vi "AI_StreamingBufferedRead.vi"(8 "error in (no error)":errorcluster, 10 "stop?":bool, 11 "Task ID":u32) -> (0 "error out":errorcluster, 1 "stopped":bool, 2 "data out":dynamicdata(graph), 3 "Task out ID":u32)   [LabVIEW 2015]
panel:
  out "status":bool
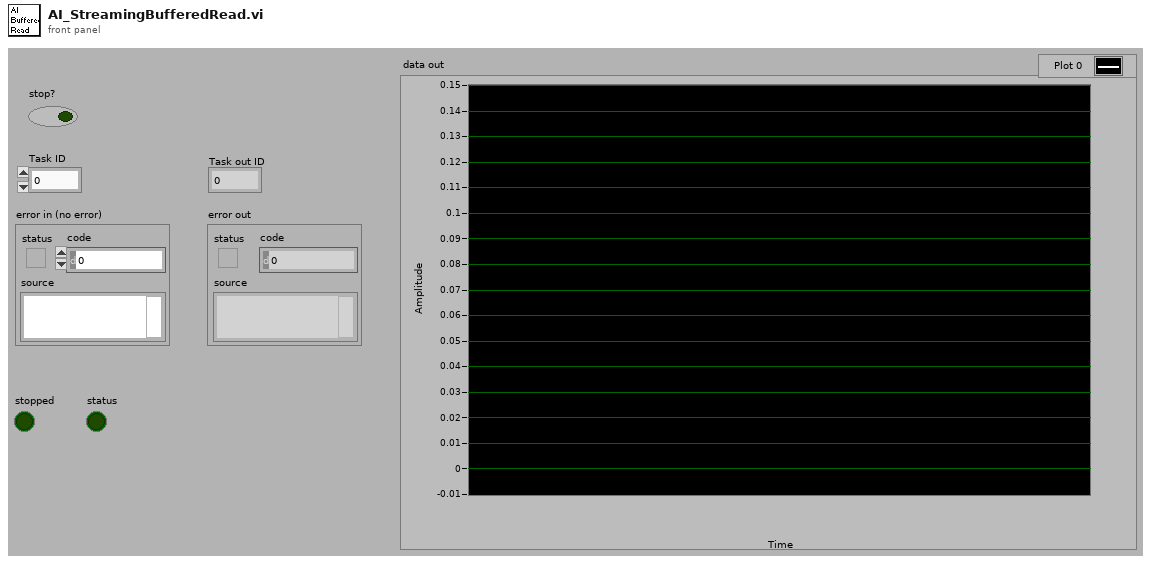
[diagram p1: front panel]
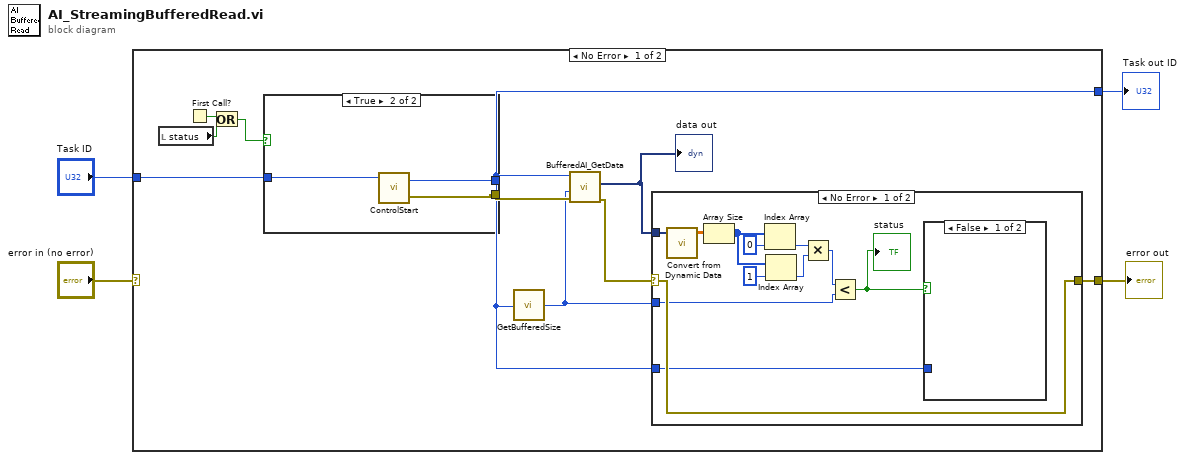
[diagram p0: block diagram]
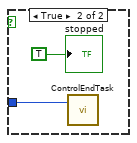
[diagram p2: hidden frame]
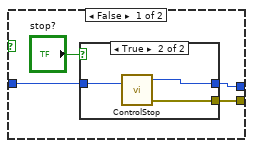
[diagram p4: hidden frame]
diagram:
  n1 = case shown="No Error" "error in (no error)" {
    selector: "error in (no error)" -> [_ w41]
    tunnel: "Task ID" -> [w14 w42]
    tunnel: [w9 w42] -> w2
    tunnel: [w12 w41] -> w1
    frame No Error {
      n2 = local read "status"() -> (w5:bool)
      n3 = First Call?() -> (First Call?: T/F=w7:bool)
      n4 = Or(x=w7, y=w5) -> (x .or. y?=w6:bool)
      n5 = case shown="True" w6 {
        tunnel: w14 -> [w33 w40]
        tunnel: [w31 w39] -> w9
        tunnel: [w30 w38] -> w10
        frame False {
          n6 = case shown="True" "stop?" {
            tunnel: w33 -> [w34 w37]
            tunnel: [w34 w36] -> w31
            tunnel: [_ w35] -> w30
            frame False {
            }
            frame True {
              n7 = call "ControlStop.vi"("Task ID"=w37) -> ("error out"=w35:errorcluster, "Task ID"=w36:u32)  [unwired: 1 in, 2 out]
            }
          }
        }
        frame True {
          n8 = call "ControlStart.vi"("Task ID"=w40) -> ("error out"=w38:errorcluster, "Task ID"=w39:u32)  [unwired: 1 in, 1 out]
        }
      }
      n9 = call "GetBufferedSize.vi"("Task ID"=w9) -> ("return type"=w8:i32)
      n10 = call "BufferedAI_GetData.vi"("error in (no error)"=w10, "count"=w8, "Task ID"=w9) -> ("error out"=w13:errorcluster, "data out"=w11:dynamicdata)  [unwired: 1 in, 6 out]
      "data out" <- w11
      n11 = case shown="No Error" w13 {
        selector: w13 -> [w25 w29]
        tunnel: [w25 w29] -> w12
        tunnel: w11 -> [w26 _]
        tunnel: w9 -> [w24 _]
        tunnel: w8 -> [w16 _]
        frame No Error {
          n12 = call "Convert from Dynamic Data"("Dynamic Data Type"=w26) -> ("Array"=w23:dbl[][])  [unwired: 3 out]
          n13 = Array Size(array=w23) -> (size(s)=w21:i32[])
          n14 = Index Array(array=w21, index=0) -> (element=w18:i32)
          n15 = Index Array(array=w21, index=1) -> (element=w19:i32)
          n16 = Multiply(x=w18, y=w19) -> (x*y=w17:i32)
          n17 = Less?(x=w17, y=w16) -> (x < y?=w15:bool)
          "status" <- w15
          n18 = case shown="False" w15 {
            tunnel: w24 -> [_ w27]
            frame False {
            }
            frame True {
              n19 = call "ControlEndTask.vi"("Task ID"=w27) -> ()  [unwired: 1 in, 2 out]
              "stopped" <- TRUE ("stopped")
            }
          }
        }
        frame Error {
        }
      }
    }
    frame Error {
    }
  }
  "Task out ID" <- w2
  "error out" <- w1
